vi "ClassPanel.vi"(8 "error in (no error)":errorcluster caption="entrée d'erreur (pas d'erreur)", 11 "Agilent34410A.lvclass":refnum<class "Agilent34410A.lvclass">) -> (0 "error out":errorcluster caption="sortie d'erreur", 3 "Agilent34410A.lvclass Out":refnum<class "Agilent34410A.lvclass">)   [LabVIEW 2019, in "Agilent34410A.lvclass"]
uses:
  Agilent34410A.lvclass
  C:/Programmes Labview/LabScanV1A/DevicesClass/BaseDevice/BaseDevice.lvclass
  <userlib>/Agilent34410A/Agilent34410A DMM_Func.ctl
  BaseDevice/Accessor/GetClassEvent.vi
panel:
  in  "NPLC":T1(ring)
  in  "Mode":enum16{"NPLC", "Apperture"}(ring)
  in  "TrigSrce":enum16{"Immediate", "External", "Bus"}(ring) caption="Trigger Source"
  in  "Aperture (s)":dbl
  in  "Autorange":bool
  in  "Range":u16(ring) items=["100 mV", "1 V", "10 V", "100 V", "1000 V", "Min", "Max", "Def"]
  in  "DMM Func":T2 caption="DMM Function"
  in  "Stop":bool
  out "Value":dbl caption="Read Value" format="%^_6e"
  in  "MiseAJour":bool
  out "Init Program":bool
  # "this MUST labeled with class name"
  # "this MUST be present and labeled \"Stop\""
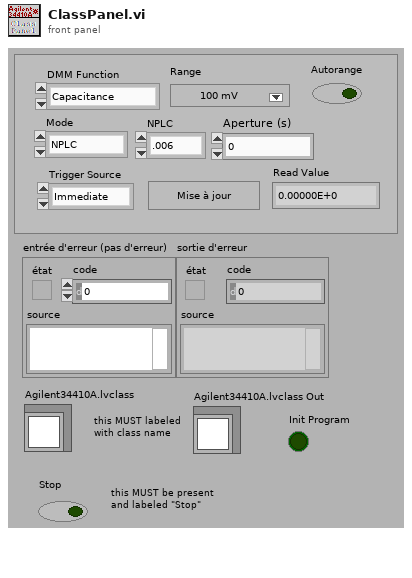
[diagram p1: front panel]
types:
  T1 = enum16{".006", ".02", ".06", ".2", "1", "2", "10", "100"}
  T2 = typedef "Agilent34410A DMM_Func.ctl" = enum16{"Capacitance", "Continuity", "Current AC", "Current", "Diode", "Frequency", "4W Resistance", "Period", "Resistance", "Temperature", "Voltage AC", "Voltage"}
  T3 = enum8{"Enabled", "Disabled", "Disabled and Grayed Out"}
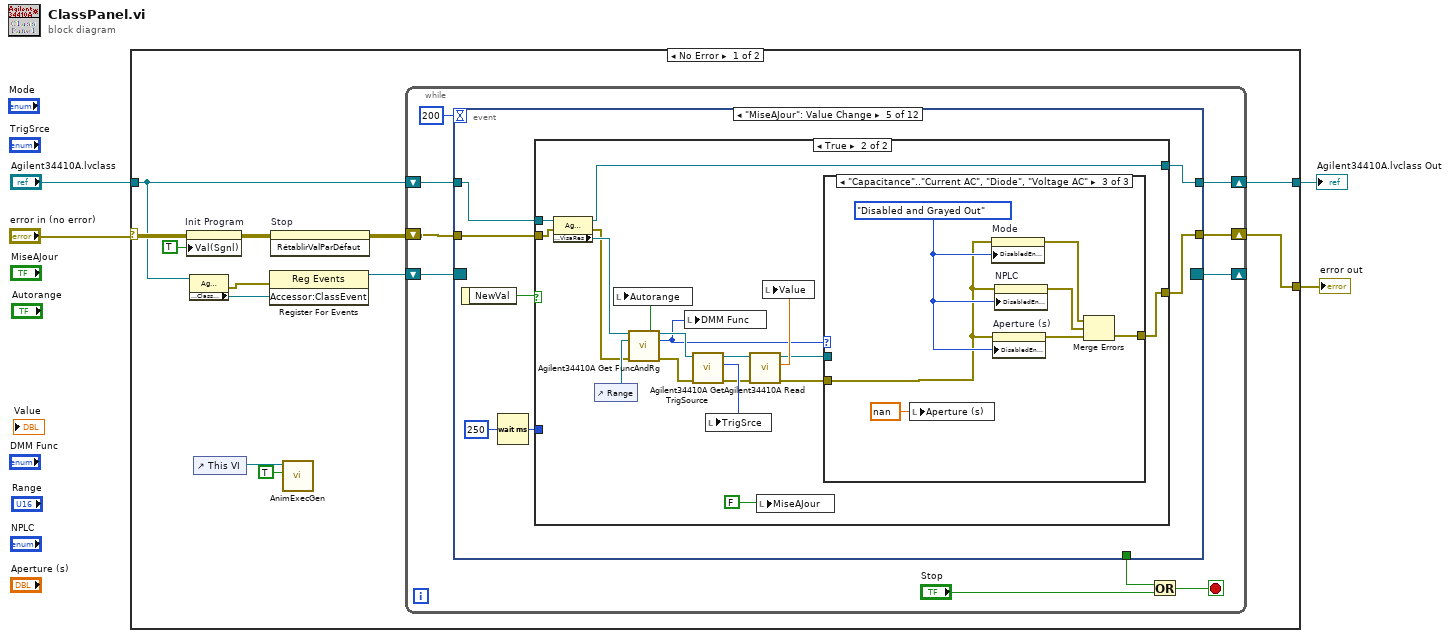
[diagram p0: block diagram]
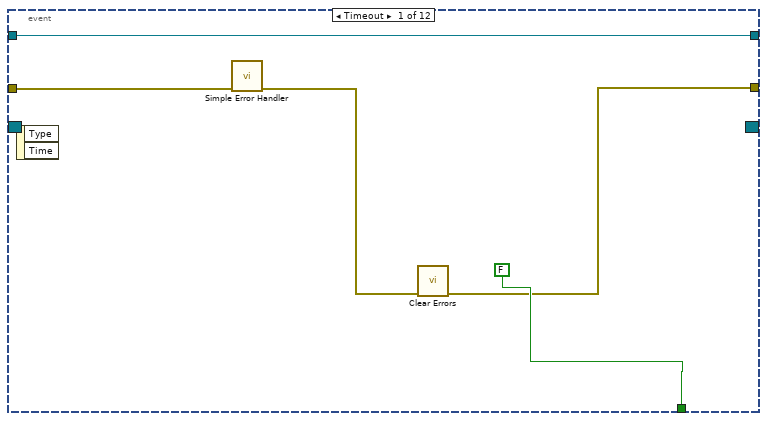
[diagram p2: hidden frame]
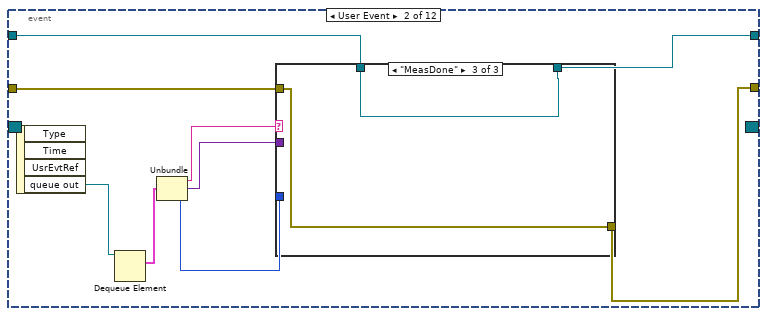
[diagram p3: hidden frame]
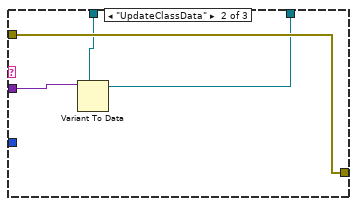
[diagram p5: hidden frame]
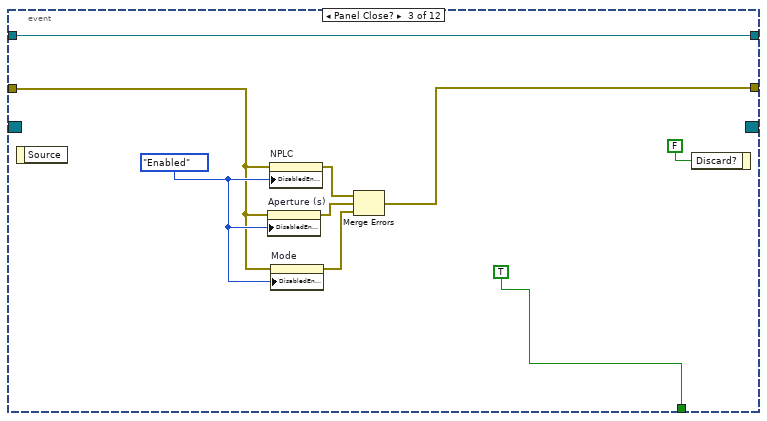
[diagram p6: hidden frame]
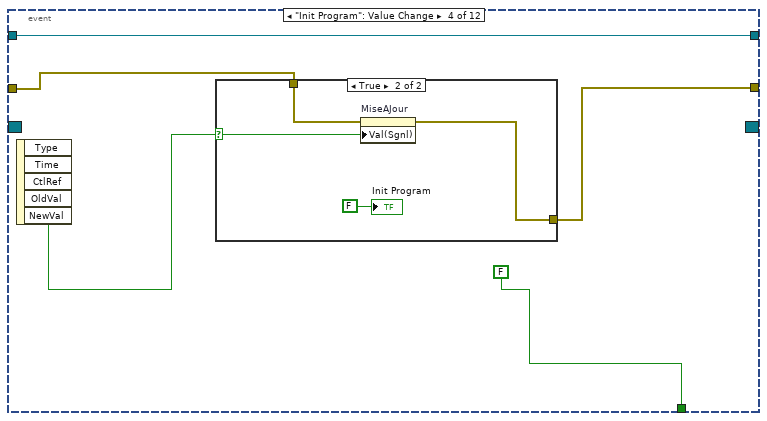
[diagram p7: hidden frame]
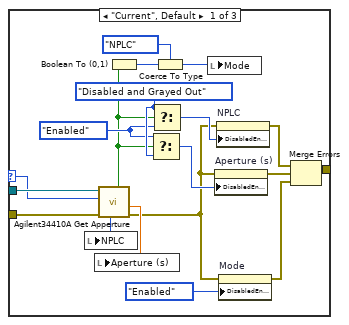
[diagram p10: hidden frame]
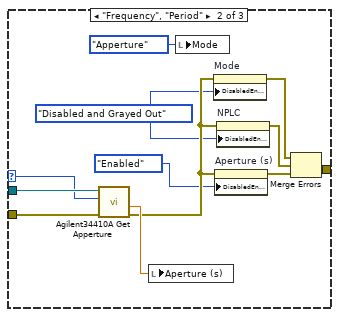
[diagram p11: hidden frame]
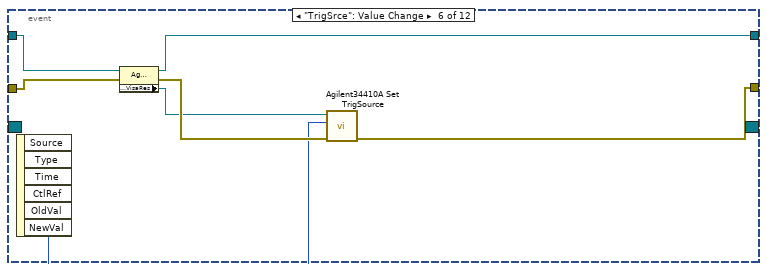
[diagram p12: hidden frame]
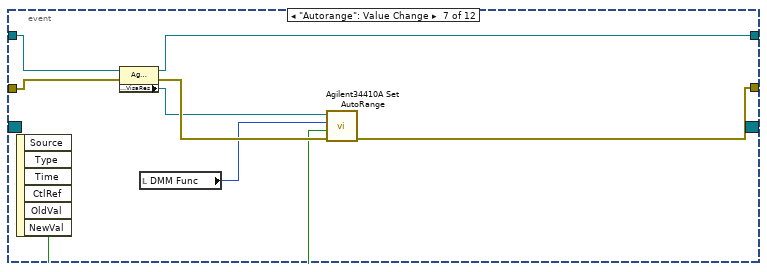
[diagram p13: hidden frame]
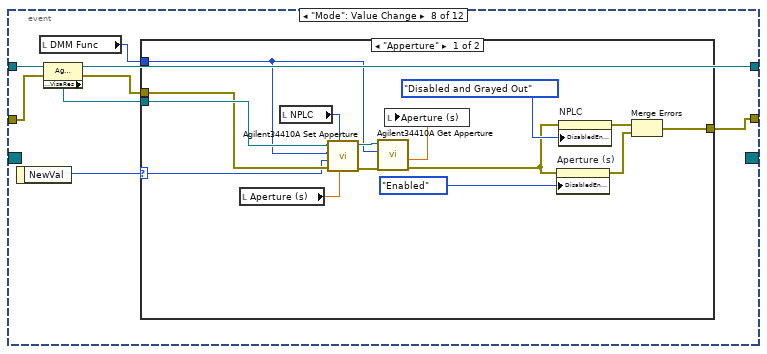
[diagram p14: hidden frame]
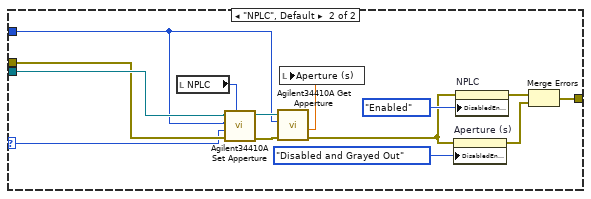
[diagram p15: hidden frame]
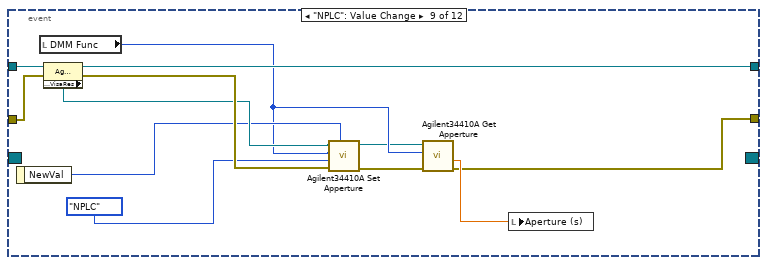
[diagram p16: hidden frame]
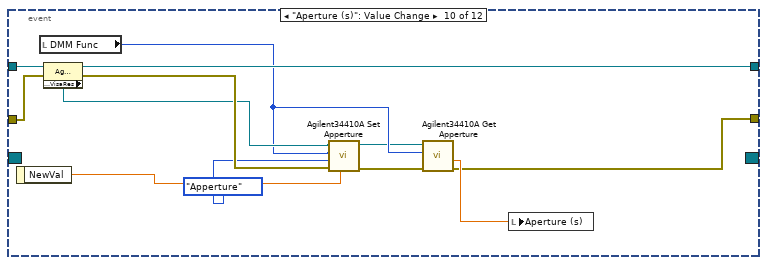
[diagram p17: hidden frame]
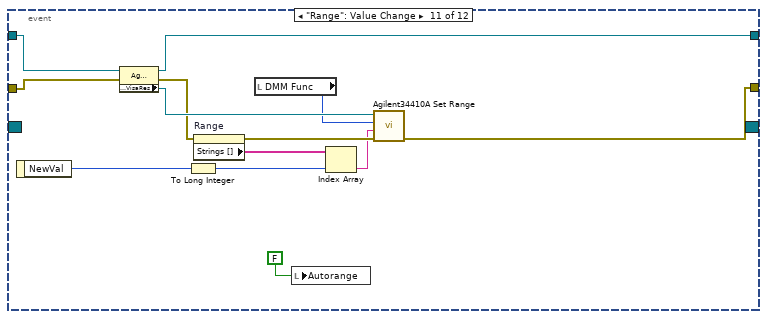
[diagram p18: hidden frame]
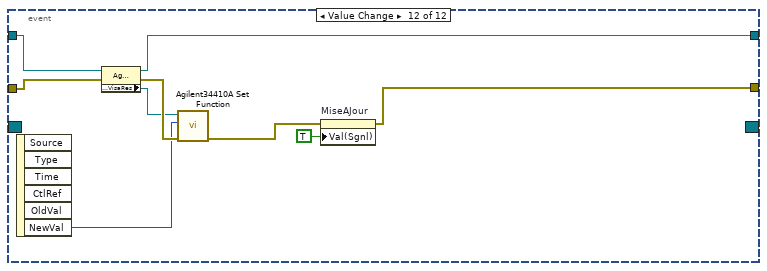
[diagram p19: hidden frame]
diagram:
  n1 = case shown="No Error" "error in (no error)" {
    selector: "error in (no error)" -> [w13 w232]
    tunnel: [w16 w232] -> w3
    tunnel: "Agilent34410A.lvclass" -> [w8 w231]
    tunnel: [w14 w231] -> w1
    frame No Error {
      n2 = property on="Init Program" class="Bool (strict)"(error in=w13, "Val(Sgnl)"=TRUE ("Valeur (Signalisation)")) -> (error out=w12:errorcluster)  [unwired: 1 in, 1 out]
      n3 = property class="Agilent34410A.lvclass"(reference=w8) -> (error out=w10:errorcluster, "Accessor:ClassEvent"=w9:refnum<user-event>)  [unwired: 1 in, 1 out]
      n4 = control-ref of="This VI"() -> (w5:refnum<vi>)
      n5 = register-events(error in=w10, w9) -> (reference out=w7:refnum<event-registration>)  [unwired: 1 in, 1 out]
      n6 = invoke on="Stop" class="Bool (strict)" method="RétablirValParDéfaut"(error in=w12) -> (error out=w11:errorcluster)  [unwired: 2 in, 2 out]
      n7 = call <userlib>:"AnimExecGen.vi"("Animer l'exécution ?"=TRUE, "ViRef"=w5) -> ()  [unwired: 9 in, 1 out]
      n8 = while {
        shift-right: [w24] -> w16
        shift-left: w11 -> [w25]
        shift-right: [w21] -> w14
        shift-left: w8 -> [w23]
        shift-right: [w17] -> _
        shift-left: w7 -> [w18]
        stop <- w20 stop-if-true
        n9 = event shown="[4] \"MiseAJour\": Value Change" {
          selector: w18 -> [_ _ _ _ _ _ _ _ _ _ _ _]
          dyn-events: [_ _ _ _ _ _ _ _ _ _ _ _] -> w17
          timeout: 200 -> [_ _ _ _ _ _ _ _ _ _ _ _]
          tunnel: w25 -> [w29 w39 w49 w61 w69 w138 w146 w154 w195 w207 w220 w229]
          tunnel: [w27 w33 w52 w60 w68 w133 w142 w148 w185 w198 w217 w223] -> w24
          tunnel: w23 -> [w30 w40 w55 w59 w71 w139 w147 w155 w196 w208 w221 w230]
          tunnel: [FALSE _ TRUE FALSE _ _ _ _ _ _ _ _] -> w22
          tunnel: [w30 w32 w55 w59 w70 w135 w143 w151 w192 w204 w218 w226] -> w21
          event Timeout {
            n10 = event-data() -> ()  [unwired: 1 in, 2 out]
            n11 = call <vilib>:"Simple Error Handler.vi"("error in (no error)"=w29) -> ("error out"=w28:errorcluster)  [unwired: 4 in, 4 out]
            n12 = call <vilib>:"Clear Errors.vi"("error in (no error)"=w28) -> ("error out"=w27:errorcluster)  [unwired: 5 in, 1 out]
          }
          event User Event {
            n13 = event-data() -> ("queue out"=w37:refnum<queue>)  [unwired: 1 in, 3 out]
            n14 = Dequeue Element(queue=w37) -> (element=w38:cluster{"Message":string, "Data":variant, i32})  [unwired: 2 in, 3 out]
            n15 = Unbundle(w38) -> ("Message"=w36:string, "Data"=w35:variant, w34:i32)
            n16 = case shown="\"MeasDone\"" w36 {
              tunnel: w39 -> [w42 w46 w47]
              tunnel: w35 -> [_ w45 _]
              tunnel: w40 -> [w41 w44 w48]
              tunnel: [w41 w43 w48] -> w32
              tunnel: [w42 w46 w47] -> w33
              tunnel: w34 -> [_ _ _]
              frame Default {
              }
              frame "UpdateClassData" {
                n17 = Variant To Data(type=w44, Variant=w45) -> (data=w43:refnum<class "Agilent34410A.lvclass">)  [unwired: 1 in, 1 out]
              }
              frame "MeasDone" {
              }
            }
          }
          event Panel Close? {
            w51 = T3."Enabled" ("Désactivé")
            n18 = event-data() -> ()  [unwired: 1 in, 1 out]
            n19 = property on="Aperture (s)" class="NumNb (strict)"(error in=w49, "DisabledEnum"=w51) -> (error out=w53:errorcluster)  [unwired: 1 in, 1 out]
            n20 = property on="NPLC" class="Énum (strict)"(error in=w49, "DisabledEnum"=w51) -> (error out=w54:errorcluster)  [unwired: 1 in, 1 out]
            n21 = property on="Mode" class="Énum (strict)"(error in=w49, "DisabledEnum"=w51) -> (error out=w50:errorcluster)  [unwired: 1 in, 1 out]
            n22 = Merge Errors(w54, w53, w50) -> (w52:errorcluster)
            n23 = event-data("Discard?"=FALSE ("Rejeter ?")) -> ()  [unwired: 1 in, 1 out]
          }
          event "Init Program": Value Change {
            n24 = event-data() -> ("NewVal"=w62:bool)  [unwired: 1 in, 4 out]
            n25 = case shown="True" w62 {
              selector: w62 -> [_ w66]
              tunnel: w61 -> [w63 w65]
              tunnel: [w63 w64] -> w60
              frame False {
              }
              frame True {
                n26 = property on="MiseAJour" class="Bool (strict)"(error in=w65, "Val(Sgnl)"=w66) -> (error out=w64:errorcluster)  [unwired: 1 in, 1 out]
                "Init Program" <- FALSE
              }
            }
          }
          event "MiseAJour": Value Change {
            n27 = event-data() -> ("NewVal"=w74:bool)  [unwired: 1 in]
            n28 = Wait (ms)(milliseconds to wait=u32 250 ("attente (ms)")) -> (millisecond timer value=w73:u32)
            n29 = case shown="True" w74 {
              tunnel: w73 -> [_ _]
              tunnel: w71 -> [w76 w93]
              tunnel: [w76 w91] -> w70
              tunnel: w69 -> [w75 w89]
              tunnel: [w75 w83] -> w68
              frame False {
              }
              frame True {
                n30 = property class="Agilent34410A.lvclass"(reference=w93, error in=w89) -> (reference out=w91:refnum<class "Agilent34410A.lvclass">, error out=w88:errorcluster, "Accessor:VisaRes"=w92:refnum<visa-resource-name>)
                n31 = control-ref of="Range"() -> (w90:refnum<vi>)
                n32 = call <userlib>:"Agilent34410A Get FuncAndRg.vi"("VISA Rsrc"=w92, "Refnum Cmde"=w90, "error in (no error)"=w88) -> ("Autorange"=w87:bool, "VISA Rsrc Out"=w85:refnum<visa-resource-name>, "DMM Function"=w81:T2, "error out"=w86:errorcluster)  [unwired: 4 in, 5 out]
                n33 = local write "Autorange"(w87) -> ()
                n34 = local write "DMM Func"(w81) -> ()
                n35 = call <userlib>:"Agilent34410A Get TrigSource.vi"("error in (no error)"=w86, "VISA Rsrc"=w85) -> ("error out"=w79:errorcluster, "Trigger Source"=w84:enum16{"Immediate", "External", "Bus"}, "VISA Rsrc Out"=w80:refnum<visa-resource-name>)  [unwired: 5 in, 2 out]
                n36 = local write "TrigSrce"(w84) -> ()
                n37 = call <userlib>:"Agilent34410A Read.vi"("error in (no error)"=w79, "VISA Rsrc"=w80) -> ("error out"=w78:errorcluster, "Reading"=w82:dbl, "VISA Rsrc Out"=w77:refnum<visa-resource-name>)  [unwired: 6 in, 1 out]
                n38 = local write "MiseAJour"(FALSE ("MiseAJour")) -> ()
                n39 = local write "Value"(w82) -> ()
                n40 = case shown="\"Capacitance\"..\"Current AC\", \"Diode\", \"Voltage AC\"" w81 {
                  selector: w81 -> [w98 w119 _]
                  tunnel: w78 -> [w113 w125 w127]
                  tunnel: w77 -> [w112 w124 _]
                  tunnel: [w104 w121 w129] -> w83
                  frame "Current", Default {
                    w107 = T3."Disabled and Grayed Out" ("Désactivé")
                    w106 = T3."Enabled" ("Désactivé")
                    n41 = call <userlib>:"Agilent34410A Get Apperture.vi"("error in (no error)"=w113, "DMM Function"=w98, "VISA Rsrc"=w112) -> ("error out"=w96:errorcluster, "Aperture (s)"=w110:dbl, "Apperture Enable"=w102:bool, "NPLC"=w111:T1)  [unwired: 2 in, 3 out]
                    n42 = local write "NPLC"(w111) -> ()
                    n43 = local write "Aperture (s)"(w110) -> ()
                    n44 = Boolean To (0,1)(Boolean=w102) -> (0, 1=w101:i16)
                    n45 = Select(t=w106, s=w102, f=w107) -> (s? t:f=w108:T3)
                    n46 = Select(t=w107, s=w102, f=w106) -> (s? t:f=w105:T3)
                    n47 = Coerce To Type(0:w101, 1:enum16{"NPLC", "Apperture"}."NPLC" ("Mode")) -> (2:w100:enum16{"NPLC", "Apperture"})
                    n48 = local write "Mode"(w100) -> ()
                    n49 = property on="Aperture (s)" class="NumNb (strict)"(error in=w96, "DisabledEnum"=w108) -> (error out=w109:errorcluster)  [unwired: 1 in, 1 out]
                    n50 = property on="NPLC" class="Énum (strict)"(error in=w96, "DisabledEnum"=w105) -> (error out=w103:errorcluster)  [unwired: 1 in, 1 out]
                    n51 = property on="Mode" class="Énum (strict)"(error in=w96, "DisabledEnum"=T3."Enabled" ("Désactivé")) -> (error out=w95:errorcluster)  [unwired: 1 in, 1 out]
                    n52 = Merge Errors(w103, w109, w95) -> (w104:errorcluster)
                  }
                  frame "Frequency", "Period" {
                    w115 = T3."Disabled and Grayed Out" ("Désactivé")
                    n53 = call <userlib>:"Agilent34410A Get Apperture.vi"("error in (no error)"=w125, "DMM Function"=w119, "VISA Rsrc"=w124) -> ("error out"=w116:errorcluster, "Aperture (s)"=w123:dbl)  [unwired: 2 in, 5 out]
                    n54 = local write "Aperture (s)"(w123) -> ()
                    n55 = local write "Mode"(enum16{"NPLC", "Apperture"}."Apperture" ("Mode")) -> ()
                    n56 = property on="Mode" class="Énum (strict)"(error in=w116, "DisabledEnum"=w115) -> (error out=w117:errorcluster)  [unwired: 1 in, 1 out]
                    n57 = property on="Aperture (s)" class="NumNb (strict)"(error in=w116, "DisabledEnum"=T3."Enabled" ("Désactivé")) -> (error out=w122:errorcluster)  [unwired: 1 in, 1 out]
                    n58 = property on="NPLC" class="Énum (strict)"(error in=w116, "DisabledEnum"=w115) -> (error out=w120:errorcluster)  [unwired: 1 in, 1 out]
                    n59 = Merge Errors(w117, w120, w122) -> (w121:errorcluster)
                  }
                  frame "Capacitance".."Current AC", "Diode", "Voltage AC" {
                    w128 = T3."Disabled and Grayed Out" ("Désactivé")
                    n60 = local write "Aperture (s)"(nan ("Aperture (s)")) -> ()
                    n61 = property on="Mode" class="Énum (strict)"(error in=w127, "DisabledEnum"=w128) -> (error out=w130:errorcluster)  [unwired: 1 in, 1 out]
                    n62 = property on="Aperture (s)" class="NumNb (strict)"(error in=w127, "DisabledEnum"=w128) -> (error out=w132:errorcluster)  [unwired: 1 in, 1 out]
                    n63 = property on="NPLC" class="Énum (strict)"(error in=w127, "DisabledEnum"=w128) -> (error out=w131:errorcluster)  [unwired: 1 in, 1 out]
                    n64 = Merge Errors(w130, w131, w132) -> (w129:errorcluster)
                  }
                }
              }
            }
          }
          event "TrigSrce": Value Change {
            n65 = event-data() -> ("NewVal"=w134:enum16{"Immediate", "External", "Bus"})  [unwired: 1 in, 5 out]
            n66 = property class="Agilent34410A.lvclass"(reference=w139, error in=w138) -> (reference out=w135:refnum<class "Agilent34410A.lvclass">, error out=w137:errorcluster, "Accessor:VisaRes"=w136:refnum<visa-resource-name>)
            n67 = call <userlib>:"Agilent34410A Set TrigSource.vi"("error in (no error)"=w137, "Trigger Source"=w134, "VISA Rsrc"=w136) -> ("error out"=w133:errorcluster)  [unwired: 6 in, 2 out]
          }
          event "Autorange": Value Change {
            n68 = event-data() -> ("NewVal"=w141:bool)  [unwired: 1 in, 5 out]
            n69 = property class="Agilent34410A.lvclass"(reference=w147, error in=w146) -> (reference out=w143:refnum<class "Agilent34410A.lvclass">, error out=w145:errorcluster, "Accessor:VisaRes"=w144:refnum<visa-resource-name>)
            n70 = local read "DMM Func"() -> (w140:T2)
            n71 = call <userlib>:"Agilent34410A Set AutoRange.vi"("error in (no error)"=w145, "AutoRange"=w141, "DMM Function"=w140, "VISA Rsrc"=w144) -> ("error out"=w142:errorcluster)  [unwired: 5 in, 2 out]
          }
          event "Mode": Value Change {
            n72 = event-data() -> ("NewVal"=w149:enum16{"NPLC", "Apperture"})  [unwired: 1 in]
            n73 = local read "DMM Func"() -> (w150:T2)
            n74 = property class="Agilent34410A.lvclass"(reference=w155, error in=w154) -> (reference out=w151:refnum<class "Agilent34410A.lvclass">, error out=w153:errorcluster, "Accessor:VisaRes"=w152:refnum<visa-resource-name>)
            n75 = case shown="\"Apperture\"" w149 {
              selector: w149 -> [w165 w180]
              tunnel: w153 -> [w169 w183]
              tunnel: w152 -> [w170 w184]
              tunnel: w150 -> [w156 w171]
              tunnel: [w162 w177] -> w148
              frame "Apperture" {
                n76 = local read "Aperture (s)"() -> (w166:dbl)
                n77 = local read "NPLC"() -> (w167:T1)
                n78 = call <userlib>:"Agilent34410A Set Apperture.vi"("Aperture (s)"=w166, "NPLC"=w167, "error in (no error)"=w169, "Mode"=w165, "DMM Function"=w156, "VISA Rsrc"=w170) -> ("error out"=w160:errorcluster, "VISA Rsrc Out"=w159:refnum<visa-resource-name>)  [unwired: 3 in, 1 out]
                n79 = call <userlib>:"Agilent34410A Get Apperture.vi"("error in (no error)"=w160, "DMM Function"=w156, "VISA Rsrc"=w159) -> ("error out"=w157:errorcluster, "Aperture (s)"=w158:dbl)  [unwired: 2 in, 5 out]
                n80 = local write "Aperture (s)"(w158) -> ()
                n81 = property on="Aperture (s)" class="NumNb (strict)"(error in=w157, "DisabledEnum"=T3."Enabled" ("Désactivé")) -> (error out=w161:errorcluster)  [unwired: 1 in, 1 out]
                n82 = property on="NPLC" class="Énum (strict)"(error in=w157, "DisabledEnum"=T3."Disabled and Grayed Out" ("Désactivé")) -> (error out=w163:errorcluster)  [unwired: 1 in, 1 out]
                n83 = Merge Errors(w163, w161) -> (w162:errorcluster)
              }
              frame "NPLC", Default {
                n84 = local read "NPLC"() -> (w181:T1)
                n85 = call <userlib>:"Agilent34410A Set Apperture.vi"("NPLC"=w181, "error in (no error)"=w183, "Mode"=w180, "DMM Function"=w171, "VISA Rsrc"=w184) -> ("error out"=w175:errorcluster, "VISA Rsrc Out"=w173:refnum<visa-resource-name>)  [unwired: 4 in, 1 out]
                n86 = call <userlib>:"Agilent34410A Get Apperture.vi"("error in (no error)"=w175, "DMM Function"=w171, "VISA Rsrc"=w173) -> ("error out"=w174:errorcluster, "Aperture (s)"=w172:dbl)  [unwired: 2 in, 5 out]
                n87 = local write "Aperture (s)"(w172) -> ()
                n88 = property on="Aperture (s)" class="NumNb (strict)"(error in=w174, "DisabledEnum"=T3."Disabled and Grayed Out" ("Désactivé")) -> (error out=w176:errorcluster)  [unwired: 1 in, 1 out]
                n89 = property on="NPLC" class="Énum (strict)"(error in=w174, "DisabledEnum"=T3."Enabled" ("Désactivé")) -> (error out=w178:errorcluster)  [unwired: 1 in, 1 out]
                n90 = Merge Errors(w178, w176) -> (w177:errorcluster)
              }
            }
          }
          event "NPLC": Value Change {
            n91 = event-data() -> ("NewVal"=w191:T1)  [unwired: 1 in]
            n92 = local read "DMM Func"() -> (w188:T2)
            n93 = property class="Agilent34410A.lvclass"(reference=w196, error in=w195) -> (reference out=w192:refnum<class "Agilent34410A.lvclass">, error out=w194:errorcluster, "Accessor:VisaRes"=w193:refnum<visa-resource-name>)
            n94 = call <userlib>:"Agilent34410A Set Apperture.vi"("NPLC"=w191, "error in (no error)"=w194, "Mode"=enum16{"NPLC", "Apperture"}."NPLC", "DMM Function"=w188, "VISA Rsrc"=w193) -> ("error out"=w189:errorcluster, "VISA Rsrc Out"=w187:refnum<visa-resource-name>)  [unwired: 4 in, 1 out]
            n95 = call <userlib>:"Agilent34410A Get Apperture.vi"("error in (no error)"=w189, "DMM Function"=w188, "VISA Rsrc"=w187) -> ("error out"=w185:errorcluster, "Aperture (s)"=w186:dbl)  [unwired: 2 in, 5 out]
            n96 = local write "Aperture (s)"(w186) -> ()
          }
          event "Aperture (s)": Value Change {
            n97 = event-data() -> ("NewVal"=w197:dbl)  [unwired: 1 in]
            n98 = local read "DMM Func"() -> (w201:T2)
            n99 = property class="Agilent34410A.lvclass"(reference=w208, error in=w207) -> (reference out=w204:refnum<class "Agilent34410A.lvclass">, error out=w206:errorcluster, "Accessor:VisaRes"=w205:refnum<visa-resource-name>)
            n100 = call <userlib>:"Agilent34410A Set Apperture.vi"("Aperture (s)"=w197, "error in (no error)"=w206, "Mode"=enum16{"NPLC", "Apperture"}."Apperture", "DMM Function"=w201, "VISA Rsrc"=w205) -> ("error out"=w202:errorcluster, "VISA Rsrc Out"=w200:refnum<visa-resource-name>)  [unwired: 4 in, 1 out]
            n101 = call <userlib>:"Agilent34410A Get Apperture.vi"("error in (no error)"=w202, "DMM Function"=w201, "VISA Rsrc"=w200) -> ("error out"=w198:errorcluster, "Aperture (s)"=w199:dbl)  [unwired: 2 in, 5 out]
            n102 = local write "Aperture (s)"(w199) -> ()
          }
          event "Range": Value Change {
            n103 = event-data() -> ("NewVal"=w212:u16)  [unwired: 1 in]
            n104 = property class="Agilent34410A.lvclass"(reference=w221, error in=w220) -> (reference out=w218:refnum<class "Agilent34410A.lvclass">, error out=w215:errorcluster, "Accessor:VisaRes"=w219:refnum<visa-resource-name>)
            n105 = To Long Integer(number=w212) -> (32bit integer=w210:i32)
            n106 = property on="Range" class="MDér (strict)"(error in=w215) -> (error out=w214:errorcluster, "Strings []"=w213:string[])  [unwired: 1 in, 1 out]
            n107 = local read "DMM Func"() -> (w216:T2)
            n108 = local write "Autorange"(FALSE ("Autorange")) -> ()
            n109 = Index Array(array=w213, index=w210) -> (element=w211:string)
            n110 = call <userlib>:"Agilent34410A Set Range.vi"("error in (no error)"=w214, "Range String"=w211, "DMM Function"=w216, "VISA Rsrc"=w219) -> ("error out"=w217:errorcluster)  [unwired: 5 in, 2 out]
          }
          event Value Change {
            n111 = event-data() -> ("NewVal"=w225:T2)  [unwired: 1 in, 5 out]
            n112 = property class="Agilent34410A.lvclass"(reference=w230, error in=w229) -> (reference out=w226:refnum<class "Agilent34410A.lvclass">, error out=w228:errorcluster, "Accessor:VisaRes"=w227:refnum<visa-resource-name>)
            n113 = call <userlib>:"Agilent34410A Set Function.vi"("error in (no error)"=w228, "DMM Function"=w225, "VISA Rsrc"=w227) -> ("error out"=w224:errorcluster)  [unwired: 6 in, 2 out]
            n114 = property on="MiseAJour" class="Bool (strict)"(error in=w224, "Val(Sgnl)"=TRUE ("Valeur (Signalisation)")) -> (error out=w223:errorcluster)  [unwired: 1 in, 1 out]
          }
        }
        n115 = Or(x=w22, y="Stop") -> (x .or. y?=w20:bool)
      }
    }
    frame Error {
    }
  }
  "error out" <- w3
  "Agilent34410A.lvclass Out" <- w1
